vi "LAB1.vi"() -> ()   [LabVIEW 2020]
panel:
  out "Volume\nIndicator":dbl=1884.9555921538758 format="%.1f"
  out "Height Indicator":dbl(slide)=6.0 scale=0.0..10.0
  in  "Height\nControl":dbl(slide)=6.0 scale=0.0..10.0
  out "Indicator 2":dbl(slide)=4.0 scale=0.0..10.0 scale format="%.1f"
  in  "Control 2":dbl(knob)=4.0 scale=0.0..10.0 scale format="%.1f"
  in  "Switch 2":bool
  out "Status 1":bool
  in  "Switch 1":bool
  in  "stop":bool
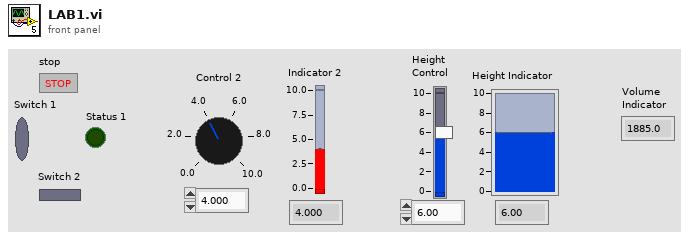
[diagram p1: front panel]
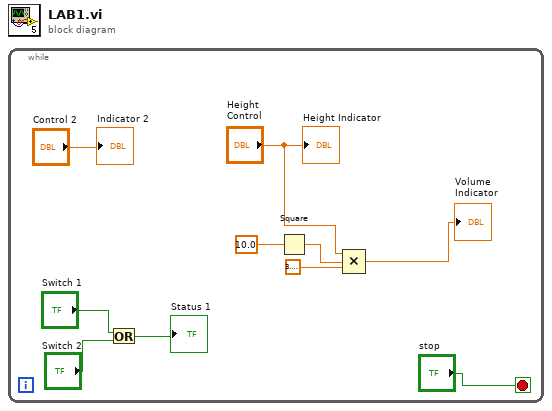
[diagram p0: block diagram]
diagram:
  n1 = while {
    stop <- "stop" stop-if-true
    n2 = Or(x="Switch 1", y="Switch 2") -> (x .or. y?=→"Status 1":bool)
    n3 = Square(x=10.0 ("result")) -> (x^2=w3:dbl)
    n4 = Compound Arithmetic op=MULTIPLY("Height\nControl", w3, 3.141592653589793) -> (→"Volume\nIndicator":dbl)
    "Indicator 2" <- "Control 2"
    "Height Indicator" <- "Height\nControl"
  }
